vi "Elevator Sensor.vi"(8 "error in":errorcluster, 10 "Value":dbl format="%#_13g", 11 "Action":T1) -> (0 "error out":errorcluster, 3 "Value":dbl)   [LabVIEW 2019]
uses:
  Typedef/FGVAction.ctl
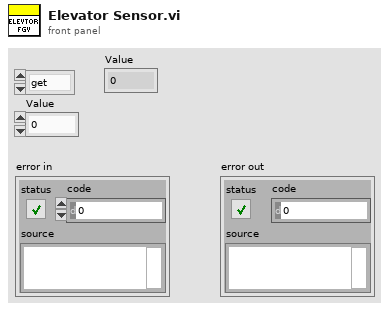
[diagram p1: front panel]
types:
  T1 = typedef "FGVAction.ctl" = enum16{"get", "set"}
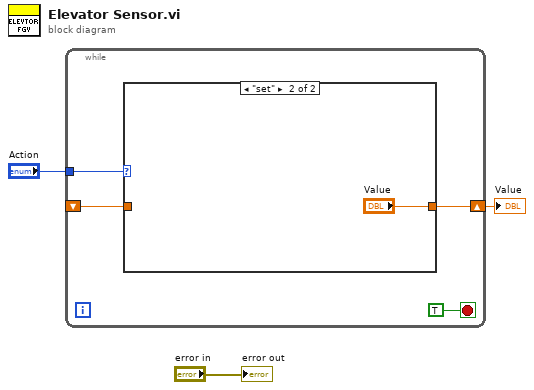
[diagram p0: block diagram]
diagram:
  n1 = while {
    tunnel: "Action" -> [w7]
    shift-right: [w6] -> w2
    shift-left: _ -> [w5]
    stop <- TRUE stop-if-true
    n2 = case shown="\"set\"" w7 {
      tunnel: [w8 "Value"] -> w6
      tunnel: w5 -> [w8 _]
      frame "get", Default {
      }
      frame "set" {
      }
    }
  }
  "Value" <- w2
  "error out" <- "error in"
